vi "Data fgv.vi"(7 "Modes":T2, 8 "error in (no error)":errorcluster, 10 "Data":T1(array[cluster])) -> (0 "error out":errorcluster, 1 "Load?":bool, 2 "Position?":bool, 3 "appended array":dbl[][](array[numeric]), 4 "Data":bool)   [LabVIEW 2016]
uses:
  Controls/data modes.ctl
  <vilib>/gmath/NI_Gmath.lvlib
panel:
  out "x-y":dbl
  out "XY Graph 2":cluster{dbl[], "yi":dbl[]}[](graph)
  out "XY Graph":cluster{dbl[], "yi":dbl[]}[](graph)
  out "Waveform Graph 4":dbl[](graph)
  out "Waveform Graph 3":dbl[](graph)
  out "Waveform Graph 2":dbl[](graph)
  out "xi used 2":dbl[](array[numeric]) format="%_6g"
  out "Array 2":dbl[](array[numeric])
  out "Waveform Graph":dbl[](graph)
  out "xi used":dbl[](array[numeric]) format="%_6g"
  out "Array":dbl[](array[numeric])
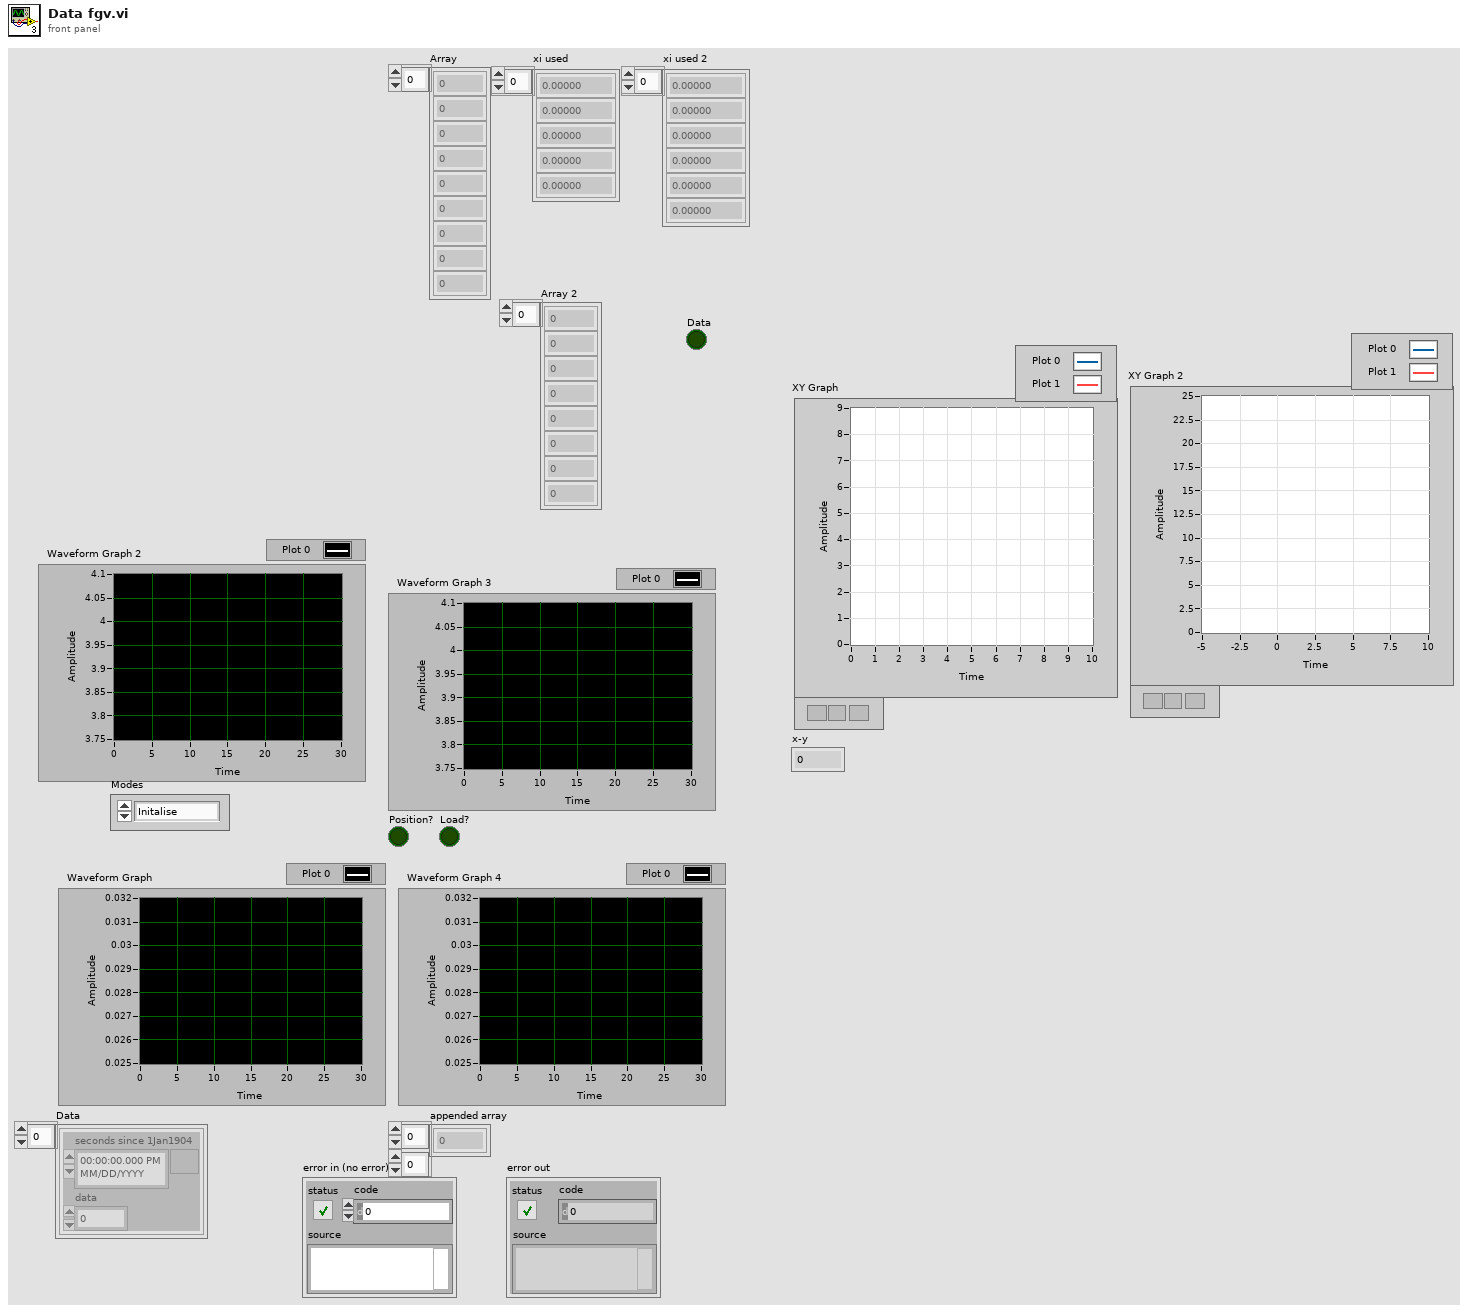
[diagram p1: front panel]
types:
  T1 = cluster{"seconds since 1Jan1904":timestamp, "data":dbl}[]
  T2 = typedef "data modes.ctl" = enum16{"Initalise", "Status", "Process", "Add load", "Add position"}
  T3 = cluster{"seconds since 1Jan1904":timestamp, "Numeric 2":dbl}[]
  T4 = cluster{"seconds since 1Jan1904":timestamp, "data":dbl}
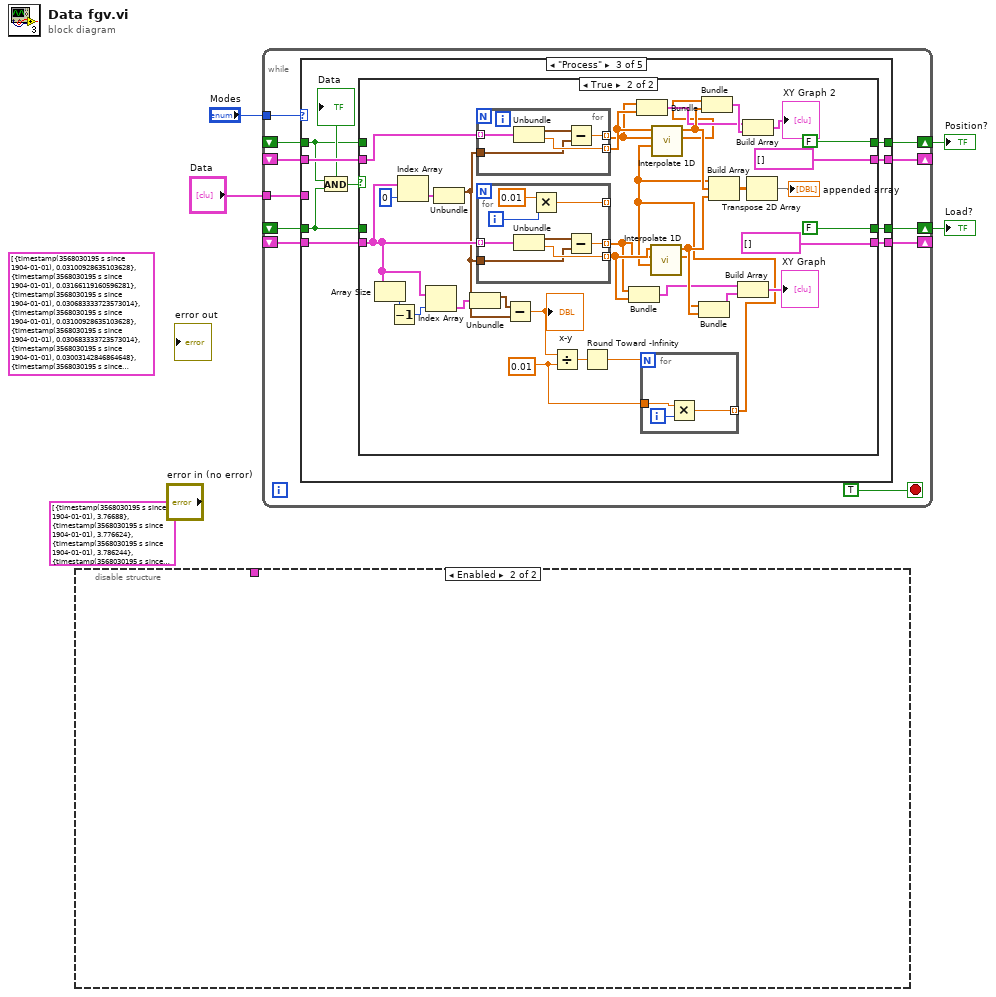
[diagram p0: block diagram]
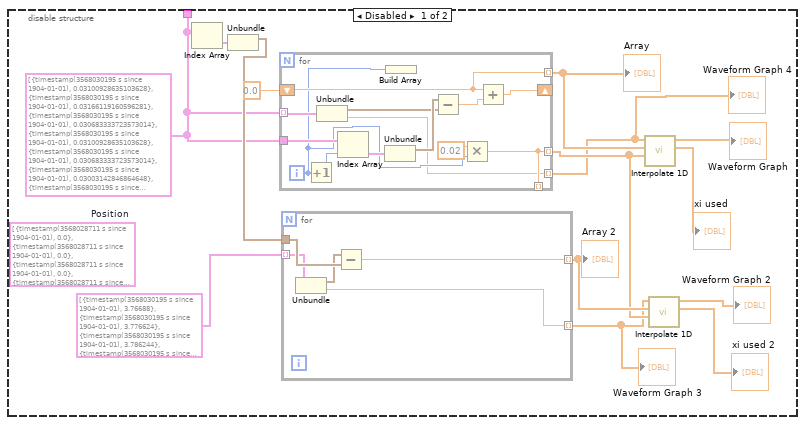
[diagram p2: hidden frame]
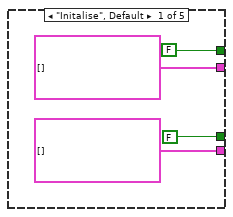
[diagram p3: hidden frame]
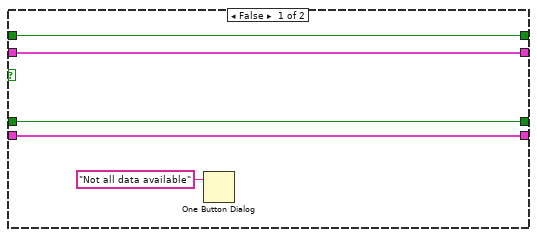
[diagram p5: hidden frame]
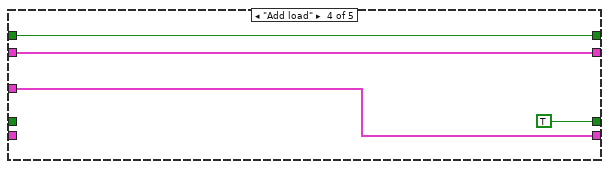
[diagram p6: hidden frame]
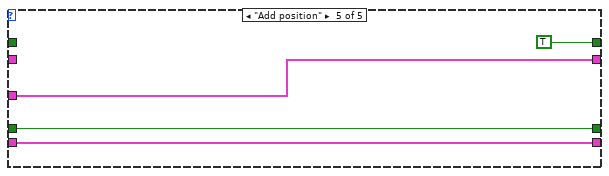
[diagram p7: hidden frame]
diagram:
  (unwired) T3 [{"seconds since 1Jan1904"=timestamp(3568030195.4029393 s since 1904-01-01), "Numeric 2"=3.76688}, {"seconds since 1Jan1904"=timestamp(3568030195.422031 s since 1904-01-01), "Numeric 2"=3.776624}, {"seconds since 1Jan1904"=timestamp(3568030195.441176 s since 1904-01-01), "Numeric 2"=3.786244}, {"seconds since 1Jan1904"=timestamp(3568030195.4632673 s since 1904-01-01), "Numeric 2"=3.796863}, {"seconds since 1Jan1904"=timestamp(3568030195.482293 s since 1904-01-01), "Numeric 2"=3.806608}, {"seconds since 1Jan1904"=timestamp(3568030195.501838 s since 1904-01-01), "Numeric 2"=3.816478}, {"seconds since 1Jan1904"=timestamp(3568030195.5218935 s since 1904-01-01), "Numeric 2"=3.826222}, {"seconds since 1Jan1904"=timestamp(3568030195.54296 s since 1904-01-01), "Numeric 2"=3.836841}, {"seconds since 1Jan1904"=timestamp(3568030195.5628576 s since 1904-01-01), "Numeric 2"=3.846836}, {"seconds since 1Jan1904"=timestamp(3568030195.582942 s since 1904-01-01), "Numeric 2"=3.85683}, {"seconds since 1Jan1904"=timestamp(3568030195.6025224 s since 1904-01-01), "Numeric 2"=3.866825}, {"seconds since 1Jan1904"=timestamp(3568030195.622336 s since 1904-01-01), "Numeric 2"=3.876445}, {"seconds since 1Jan1904"=timestamp(3568030195.642922 s since 1904-01-01), "Numeric 2"=3.886939}, {"seconds since 1Jan1904"=timestamp(3568030195.6669855 s since 1904-01-01), "Numeric 2"=3.898807}, {"seconds since 1Jan1904"=timestamp(3568030195.6822724 s since 1904-01-01), "Numeric 2"=3.906678}, {"seconds since 1Jan1904"=timestamp(3568030195.702325 s since 1904-01-01), "Numeric 2"=3.916672}, {"seconds since 1Jan1904"=timestamp(3568030195.72194 s since 1904-01-01), "Numeric 2"=3.926292}, {"seconds since 1Jan1904"=timestamp(3568030195.7419944 s since 1904-01-01), "Numeric 2"=3.936287}, {"seconds since 1Jan1904"=timestamp(3568030195.7638783 s since 1904-01-01), "Numeric 2"=3.947156}, {"seconds since 1Jan1904"=timestamp(3568030195.7819915 s since 1904-01-01), "Numeric 2"=3.956276}, {"seconds since 1Jan1904"=timestamp(3568030195.8025956 s since 1904-01-01), "Numeric 2"=3.966645}, {"seconds since 1Jan1904"=timestamp(3568030195.8226495 s since 1904-01-01), "Numeric 2"=3.976515}, {"seconds since 1Jan1904"=timestamp(3568030195.842401 s since 1904-01-01), "Numeric 2"=3.986509}, {"seconds since 1Jan1904"=timestamp(3568030195.862955 s since 1904-01-01), "Numeric 2"=3.996629}, {"seconds since 1Jan1904"=timestamp(3568030195.88289 s since 1904-01-01), "Numeric 2"=4.006748}, {"seconds since 1Jan1904"=timestamp(3568030195.9019513 s since 1904-01-01), "Numeric 2"=4.016368}, {"seconds since 1Jan1904"=timestamp(3568030195.9225645 s since 1904-01-01), "Numeric 2"=4.026487}, {"seconds since 1Jan1904"=timestamp(3568030195.942545 s since 1904-01-01), "Numeric 2"=4.036732}, {"seconds since 1Jan1904"=timestamp(3568030195.9630976 s since 1904-01-01), "Numeric 2"=4.046851}, {"seconds since 1Jan1904"=timestamp(3568030195.98266 s since 1904-01-01), "Numeric 2"=4.056471}] ("Array 3")
  (unwired) T1 [{"seconds since 1Jan1904"=timestamp(3568030195.391982 s since 1904-01-01), "data"=0.03100928635103628}, {"seconds since 1Jan1904"=timestamp(3568030195.4114995 s since 1904-01-01), "data"=0.03166119160596281}, {"seconds since 1Jan1904"=timestamp(3568030195.4307785 s since 1904-01-01), "data"=0.030683333723573014}, {"seconds since 1Jan1904"=timestamp(3568030195.4522047 s since 1904-01-01), "data"=0.03100928635103628}, {"seconds since 1Jan1904"=timestamp(3568030195.4717565 s since 1904-01-01), "data"=0.030683333723573014}, {"seconds since 1Jan1904"=timestamp(3568030195.4913096 s since 1904-01-01), "data"=0.03003142846864648}, {"seconds since 1Jan1904"=timestamp(3568030195.5108614 s since 1904-01-01), "data"=0.029705475841183215}, {"seconds since 1Jan1904"=timestamp(3568030195.5319176 s since 1904-01-01), "data"=0.02937952321371995}, {"seconds since 1Jan1904"=timestamp(3568030195.5513153 s since 1904-01-01), "data"=0.030357381096109748}, {"seconds since 1Jan1904"=timestamp(3568030195.5719137 s since 1904-01-01), "data"=0.029705475841183215}, {"seconds since 1Jan1904"=timestamp(3568030195.591967 s since 1904-01-01), "data"=0.029705475841183215}, {"seconds since 1Jan1904"=timestamp(3568030195.611306 s since 1904-01-01), "data"=0.02937952321371995}, {"seconds since 1Jan1904"=timestamp(3568030195.631862 s since 1904-01-01), "data"=0.02840166533133015}, {"seconds since 1Jan1904"=timestamp(3568030195.6559243 s since 1904-01-01), "data"=0.02937952321371995}, {"seconds since 1Jan1904"=timestamp(3568030195.671742 s since 1904-01-01), "data"=0.028075712703866884}, {"seconds since 1Jan1904"=timestamp(3568030195.6917977 s since 1904-01-01), "data"=0.02840166533133015}, {"seconds since 1Jan1904"=timestamp(3568030195.711027 s since 1904-01-01), "data"=0.027749760076403618}, {"seconds since 1Jan1904"=timestamp(3568030195.730965 s since 1904-01-01), "data"=0.027749760076403618}, {"seconds since 1Jan1904"=timestamp(3568030195.7527533 s since 1904-01-01), "data"=0.027749760076403618}, {"seconds since 1Jan1904"=timestamp(3568030195.771014 s since 1904-01-01), "data"=0.027749760076403618}, {"seconds since 1Jan1904"=timestamp(3568030195.791657 s since 1904-01-01), "data"=0.02677190219401382}, {"seconds since 1Jan1904"=timestamp(3568030195.811627 s since 1904-01-01), "data"=0.027097854821477085}, {"seconds since 1Jan1904"=timestamp(3568030195.831372 s since 1904-01-01), "data"=0.027749760076403618}, {"seconds since 1Jan1904"=timestamp(3568030195.850931 s since 1904-01-01), "data"=0.026445949566550553}, {"seconds since 1Jan1904"=timestamp(3568030195.8718615 s since 1904-01-01), "data"=0.02677190219401382}, {"seconds since 1Jan1904"=timestamp(3568030195.8914046 s since 1904-01-01), "data"=0.026445949566550553}, {"seconds since 1Jan1904"=timestamp(3568030195.911457 s since 1904-01-01), "data"=0.026119996939087287}, {"seconds since 1Jan1904"=timestamp(3568030195.9320126 s since 1904-01-01), "data"=0.025142139056697488}, {"seconds since 1Jan1904"=timestamp(3568030195.952068 s since 1904-01-01), "data"=0.02579404431162402}, {"seconds since 1Jan1904"=timestamp(3568030195.9716344 s since 1904-01-01), "data"=0.025468091684160754}] ("appended array")
  n1 = disable-structure shown="Enabled" {
    disable-tunnel: [w5 _] -> _
    frame Disabled {
      (unwired) T3 [{"seconds since 1Jan1904"=timestamp(3568030195.4029393 s since 1904-01-01), "Numeric 2"=3.76688}, {"seconds since 1Jan1904"=timestamp(3568030195.422031 s since 1904-01-01), "Numeric 2"=3.776624}, {"seconds since 1Jan1904"=timestamp(3568030195.441176 s since 1904-01-01), "Numeric 2"=3.786244}, {"seconds since 1Jan1904"=timestamp(3568030195.4632673 s since 1904-01-01), "Numeric 2"=3.796863}, {"seconds since 1Jan1904"=timestamp(3568030195.482293 s since 1904-01-01), "Numeric 2"=3.806608}, {"seconds since 1Jan1904"=timestamp(3568030195.501838 s since 1904-01-01), "Numeric 2"=3.816478}, {"seconds since 1Jan1904"=timestamp(3568030195.5218935 s since 1904-01-01), "Numeric 2"=3.826222}, {"seconds since 1Jan1904"=timestamp(3568030195.54296 s since 1904-01-01), "Numeric 2"=3.836841}, {"seconds since 1Jan1904"=timestamp(3568030195.5628576 s since 1904-01-01), "Numeric 2"=3.846836}, {"seconds since 1Jan1904"=timestamp(3568030195.582942 s since 1904-01-01), "Numeric 2"=3.85683}, {"seconds since 1Jan1904"=timestamp(3568030195.6025224 s since 1904-01-01), "Numeric 2"=3.866825}, {"seconds since 1Jan1904"=timestamp(3568030195.622336 s since 1904-01-01), "Numeric 2"=3.876445}, {"seconds since 1Jan1904"=timestamp(3568030195.642922 s since 1904-01-01), "Numeric 2"=3.886939}, {"seconds since 1Jan1904"=timestamp(3568030195.6669855 s since 1904-01-01), "Numeric 2"=3.898807}, {"seconds since 1Jan1904"=timestamp(3568030195.6822724 s since 1904-01-01), "Numeric 2"=3.906678}, {"seconds since 1Jan1904"=timestamp(3568030195.702325 s since 1904-01-01), "Numeric 2"=3.916672}, {"seconds since 1Jan1904"=timestamp(3568030195.72194 s since 1904-01-01), "Numeric 2"=3.926292}, {"seconds since 1Jan1904"=timestamp(3568030195.7419944 s since 1904-01-01), "Numeric 2"=3.936287}, {"seconds since 1Jan1904"=timestamp(3568030195.7638783 s since 1904-01-01), "Numeric 2"=3.947156}, {"seconds since 1Jan1904"=timestamp(3568030195.7819915 s since 1904-01-01), "Numeric 2"=3.956276}, {"seconds since 1Jan1904"=timestamp(3568030195.8025956 s since 1904-01-01), "Numeric 2"=3.966645}, {"seconds since 1Jan1904"=timestamp(3568030195.8226495 s since 1904-01-01), "Numeric 2"=3.976515}, {"seconds since 1Jan1904"=timestamp(3568030195.842401 s since 1904-01-01), "Numeric 2"=3.986509}, {"seconds since 1Jan1904"=timestamp(3568030195.862955 s since 1904-01-01), "Numeric 2"=3.996629}, {"seconds since 1Jan1904"=timestamp(3568030195.88289 s since 1904-01-01), "Numeric 2"=4.006748}, {"seconds since 1Jan1904"=timestamp(3568030195.9019513 s since 1904-01-01), "Numeric 2"=4.016368}, {"seconds since 1Jan1904"=timestamp(3568030195.9225645 s since 1904-01-01), "Numeric 2"=4.026487}, {"seconds since 1Jan1904"=timestamp(3568030195.942545 s since 1904-01-01), "Numeric 2"=4.036732}, {"seconds since 1Jan1904"=timestamp(3568030195.9630976 s since 1904-01-01), "Numeric 2"=4.046851}, {"seconds since 1Jan1904"=timestamp(3568030195.98266 s since 1904-01-01), "Numeric 2"=4.056471}] ("Array 3")
      (unwired) T3 [{"seconds since 1Jan1904"=timestamp(3568030195.4029393 s since 1904-01-01), "Numeric 2"=3.76688}, {"seconds since 1Jan1904"=timestamp(3568030195.422031 s since 1904-01-01), "Numeric 2"=3.776624}, {"seconds since 1Jan1904"=timestamp(3568030195.441176 s since 1904-01-01), "Numeric 2"=3.786244}, {"seconds since 1Jan1904"=timestamp(3568030195.4632673 s since 1904-01-01), "Numeric 2"=3.796863}, {"seconds since 1Jan1904"=timestamp(3568030195.482293 s since 1904-01-01), "Numeric 2"=3.806608}, {"seconds since 1Jan1904"=timestamp(3568030195.501838 s since 1904-01-01), "Numeric 2"=3.816478}, {"seconds since 1Jan1904"=timestamp(3568030195.5218935 s since 1904-01-01), "Numeric 2"=3.826222}, {"seconds since 1Jan1904"=timestamp(3568030195.54296 s since 1904-01-01), "Numeric 2"=3.836841}, {"seconds since 1Jan1904"=timestamp(3568030195.5628576 s since 1904-01-01), "Numeric 2"=3.846836}, {"seconds since 1Jan1904"=timestamp(3568030195.582942 s since 1904-01-01), "Numeric 2"=3.85683}, {"seconds since 1Jan1904"=timestamp(3568030195.6025224 s since 1904-01-01), "Numeric 2"=3.866825}, {"seconds since 1Jan1904"=timestamp(3568030195.622336 s since 1904-01-01), "Numeric 2"=3.876445}, {"seconds since 1Jan1904"=timestamp(3568030195.642922 s since 1904-01-01), "Numeric 2"=3.886939}, {"seconds since 1Jan1904"=timestamp(3568030195.6669855 s since 1904-01-01), "Numeric 2"=3.898807}, {"seconds since 1Jan1904"=timestamp(3568030195.6822724 s since 1904-01-01), "Numeric 2"=3.906678}, {"seconds since 1Jan1904"=timestamp(3568030195.702325 s since 1904-01-01), "Numeric 2"=3.916672}, {"seconds since 1Jan1904"=timestamp(3568030195.72194 s since 1904-01-01), "Numeric 2"=3.926292}, {"seconds since 1Jan1904"=timestamp(3568030195.7419944 s since 1904-01-01), "Numeric 2"=3.936287}, {"seconds since 1Jan1904"=timestamp(3568030195.7638783 s since 1904-01-01), "Numeric 2"=3.947156}, {"seconds since 1Jan1904"=timestamp(3568030195.7819915 s since 1904-01-01), "Numeric 2"=3.956276}, {"seconds since 1Jan1904"=timestamp(3568030195.8025956 s since 1904-01-01), "Numeric 2"=3.966645}, {"seconds since 1Jan1904"=timestamp(3568030195.8226495 s since 1904-01-01), "Numeric 2"=3.976515}, {"seconds since 1Jan1904"=timestamp(3568030195.842401 s since 1904-01-01), "Numeric 2"=3.986509}, {"seconds since 1Jan1904"=timestamp(3568030195.862955 s since 1904-01-01), "Numeric 2"=3.996629}, {"seconds since 1Jan1904"=timestamp(3568030195.88289 s since 1904-01-01), "Numeric 2"=4.006748}, {"seconds since 1Jan1904"=timestamp(3568030195.9019513 s since 1904-01-01), "Numeric 2"=4.016368}, {"seconds since 1Jan1904"=timestamp(3568030195.9225645 s since 1904-01-01), "Numeric 2"=4.026487}, {"seconds since 1Jan1904"=timestamp(3568030195.942545 s since 1904-01-01), "Numeric 2"=4.036732}, {"seconds since 1Jan1904"=timestamp(3568030195.9630976 s since 1904-01-01), "Numeric 2"=4.046851}, {"seconds since 1Jan1904"=timestamp(3568030195.98266 s since 1904-01-01), "Numeric 2"=4.056471}] ("Array 3")
      (unwired) T3 [{"seconds since 1Jan1904"=timestamp(3568030195.4029393 s since 1904-01-01), "Numeric 2"=3.76688}, {"seconds since 1Jan1904"=timestamp(3568030195.422031 s since 1904-01-01), "Numeric 2"=3.776624}, {"seconds since 1Jan1904"=timestamp(3568030195.441176 s since 1904-01-01), "Numeric 2"=3.786244}, {"seconds since 1Jan1904"=timestamp(3568030195.4632673 s since 1904-01-01), "Numeric 2"=3.796863}, {"seconds since 1Jan1904"=timestamp(3568030195.482293 s since 1904-01-01), "Numeric 2"=3.806608}, {"seconds since 1Jan1904"=timestamp(3568030195.501838 s since 1904-01-01), "Numeric 2"=3.816478}, {"seconds since 1Jan1904"=timestamp(3568030195.5218935 s since 1904-01-01), "Numeric 2"=3.826222}, {"seconds since 1Jan1904"=timestamp(3568030195.54296 s since 1904-01-01), "Numeric 2"=3.836841}, {"seconds since 1Jan1904"=timestamp(3568030195.5628576 s since 1904-01-01), "Numeric 2"=3.846836}, {"seconds since 1Jan1904"=timestamp(3568030195.582942 s since 1904-01-01), "Numeric 2"=3.85683}, {"seconds since 1Jan1904"=timestamp(3568030195.6025224 s since 1904-01-01), "Numeric 2"=3.866825}, {"seconds since 1Jan1904"=timestamp(3568030195.622336 s since 1904-01-01), "Numeric 2"=3.876445}, {"seconds since 1Jan1904"=timestamp(3568030195.642922 s since 1904-01-01), "Numeric 2"=3.886939}, {"seconds since 1Jan1904"=timestamp(3568030195.6669855 s since 1904-01-01), "Numeric 2"=3.898807}, {"seconds since 1Jan1904"=timestamp(3568030195.6822724 s since 1904-01-01), "Numeric 2"=3.906678}, {"seconds since 1Jan1904"=timestamp(3568030195.702325 s since 1904-01-01), "Numeric 2"=3.916672}, {"seconds since 1Jan1904"=timestamp(3568030195.72194 s since 1904-01-01), "Numeric 2"=3.926292}, {"seconds since 1Jan1904"=timestamp(3568030195.7419944 s since 1904-01-01), "Numeric 2"=3.936287}, {"seconds since 1Jan1904"=timestamp(3568030195.7638783 s since 1904-01-01), "Numeric 2"=3.947156}, {"seconds since 1Jan1904"=timestamp(3568030195.7819915 s since 1904-01-01), "Numeric 2"=3.956276}, {"seconds since 1Jan1904"=timestamp(3568030195.8025956 s since 1904-01-01), "Numeric 2"=3.966645}, {"seconds since 1Jan1904"=timestamp(3568030195.8226495 s since 1904-01-01), "Numeric 2"=3.976515}, {"seconds since 1Jan1904"=timestamp(3568030195.842401 s since 1904-01-01), "Numeric 2"=3.986509}, {"seconds since 1Jan1904"=timestamp(3568030195.862955 s since 1904-01-01), "Numeric 2"=3.996629}, {"seconds since 1Jan1904"=timestamp(3568030195.88289 s since 1904-01-01), "Numeric 2"=4.006748}, {"seconds since 1Jan1904"=timestamp(3568030195.9019513 s since 1904-01-01), "Numeric 2"=4.016368}, {"seconds since 1Jan1904"=timestamp(3568030195.9225645 s since 1904-01-01), "Numeric 2"=4.026487}, {"seconds since 1Jan1904"=timestamp(3568030195.942545 s since 1904-01-01), "Numeric 2"=4.036732}, {"seconds since 1Jan1904"=timestamp(3568030195.9630976 s since 1904-01-01), "Numeric 2"=4.046851}, {"seconds since 1Jan1904"=timestamp(3568030195.98266 s since 1904-01-01), "Numeric 2"=4.056471}] ("Array 3")
      (unwired) T3 [{"seconds since 1Jan1904"=timestamp(3568030195.4029393 s since 1904-01-01), "Numeric 2"=3.76688}, {"seconds since 1Jan1904"=timestamp(3568030195.422031 s since 1904-01-01), "Numeric 2"=3.776624}, {"seconds since 1Jan1904"=timestamp(3568030195.441176 s since 1904-01-01), "Numeric 2"=3.786244}, {"seconds since 1Jan1904"=timestamp(3568030195.4632673 s since 1904-01-01), "Numeric 2"=3.796863}, {"seconds since 1Jan1904"=timestamp(3568030195.482293 s since 1904-01-01), "Numeric 2"=3.806608}, {"seconds since 1Jan1904"=timestamp(3568030195.501838 s since 1904-01-01), "Numeric 2"=3.816478}, {"seconds since 1Jan1904"=timestamp(3568030195.5218935 s since 1904-01-01), "Numeric 2"=3.826222}, {"seconds since 1Jan1904"=timestamp(3568030195.54296 s since 1904-01-01), "Numeric 2"=3.836841}, {"seconds since 1Jan1904"=timestamp(3568030195.5628576 s since 1904-01-01), "Numeric 2"=3.846836}, {"seconds since 1Jan1904"=timestamp(3568030195.582942 s since 1904-01-01), "Numeric 2"=3.85683}, {"seconds since 1Jan1904"=timestamp(3568030195.6025224 s since 1904-01-01), "Numeric 2"=3.866825}, {"seconds since 1Jan1904"=timestamp(3568030195.622336 s since 1904-01-01), "Numeric 2"=3.876445}, {"seconds since 1Jan1904"=timestamp(3568030195.642922 s since 1904-01-01), "Numeric 2"=3.886939}, {"seconds since 1Jan1904"=timestamp(3568030195.6669855 s since 1904-01-01), "Numeric 2"=3.898807}, {"seconds since 1Jan1904"=timestamp(3568030195.6822724 s since 1904-01-01), "Numeric 2"=3.906678}, {"seconds since 1Jan1904"=timestamp(3568030195.702325 s since 1904-01-01), "Numeric 2"=3.916672}, {"seconds since 1Jan1904"=timestamp(3568030195.72194 s since 1904-01-01), "Numeric 2"=3.926292}, {"seconds since 1Jan1904"=timestamp(3568030195.7419944 s since 1904-01-01), "Numeric 2"=3.936287}, {"seconds since 1Jan1904"=timestamp(3568030195.7638783 s since 1904-01-01), "Numeric 2"=3.947156}, {"seconds since 1Jan1904"=timestamp(3568030195.7819915 s since 1904-01-01), "Numeric 2"=3.956276}, {"seconds since 1Jan1904"=timestamp(3568030195.8025956 s since 1904-01-01), "Numeric 2"=3.966645}, {"seconds since 1Jan1904"=timestamp(3568030195.8226495 s since 1904-01-01), "Numeric 2"=3.976515}, {"seconds since 1Jan1904"=timestamp(3568030195.842401 s since 1904-01-01), "Numeric 2"=3.986509}, {"seconds since 1Jan1904"=timestamp(3568030195.862955 s since 1904-01-01), "Numeric 2"=3.996629}, {"seconds since 1Jan1904"=timestamp(3568030195.88289 s since 1904-01-01), "Numeric 2"=4.006748}, {"seconds since 1Jan1904"=timestamp(3568030195.9019513 s since 1904-01-01), "Numeric 2"=4.016368}, {"seconds since 1Jan1904"=timestamp(3568030195.9225645 s since 1904-01-01), "Numeric 2"=4.026487}, {"seconds since 1Jan1904"=timestamp(3568030195.942545 s since 1904-01-01), "Numeric 2"=4.036732}, {"seconds since 1Jan1904"=timestamp(3568030195.9630976 s since 1904-01-01), "Numeric 2"=4.046851}, {"seconds since 1Jan1904"=timestamp(3568030195.98266 s since 1904-01-01), "Numeric 2"=4.056471}] ("Array 3")
      (unwired) T3 [{"seconds since 1Jan1904"=timestamp(3568030195.4029393 s since 1904-01-01), "Numeric 2"=3.76688}, {"seconds since 1Jan1904"=timestamp(3568030195.422031 s since 1904-01-01), "Numeric 2"=3.776624}, {"seconds since 1Jan1904"=timestamp(3568030195.441176 s since 1904-01-01), "Numeric 2"=3.786244}, {"seconds since 1Jan1904"=timestamp(3568030195.4632673 s since 1904-01-01), "Numeric 2"=3.796863}, {"seconds since 1Jan1904"=timestamp(3568030195.482293 s since 1904-01-01), "Numeric 2"=3.806608}, {"seconds since 1Jan1904"=timestamp(3568030195.501838 s since 1904-01-01), "Numeric 2"=3.816478}, {"seconds since 1Jan1904"=timestamp(3568030195.5218935 s since 1904-01-01), "Numeric 2"=3.826222}, {"seconds since 1Jan1904"=timestamp(3568030195.54296 s since 1904-01-01), "Numeric 2"=3.836841}, {"seconds since 1Jan1904"=timestamp(3568030195.5628576 s since 1904-01-01), "Numeric 2"=3.846836}, {"seconds since 1Jan1904"=timestamp(3568030195.582942 s since 1904-01-01), "Numeric 2"=3.85683}, {"seconds since 1Jan1904"=timestamp(3568030195.6025224 s since 1904-01-01), "Numeric 2"=3.866825}, {"seconds since 1Jan1904"=timestamp(3568030195.622336 s since 1904-01-01), "Numeric 2"=3.876445}, {"seconds since 1Jan1904"=timestamp(3568030195.642922 s since 1904-01-01), "Numeric 2"=3.886939}, {"seconds since 1Jan1904"=timestamp(3568030195.6669855 s since 1904-01-01), "Numeric 2"=3.898807}, {"seconds since 1Jan1904"=timestamp(3568030195.6822724 s since 1904-01-01), "Numeric 2"=3.906678}, {"seconds since 1Jan1904"=timestamp(3568030195.702325 s since 1904-01-01), "Numeric 2"=3.916672}, {"seconds since 1Jan1904"=timestamp(3568030195.72194 s since 1904-01-01), "Numeric 2"=3.926292}, {"seconds since 1Jan1904"=timestamp(3568030195.7419944 s since 1904-01-01), "Numeric 2"=3.936287}, {"seconds since 1Jan1904"=timestamp(3568030195.7638783 s since 1904-01-01), "Numeric 2"=3.947156}, {"seconds since 1Jan1904"=timestamp(3568030195.7819915 s since 1904-01-01), "Numeric 2"=3.956276}, {"seconds since 1Jan1904"=timestamp(3568030195.8025956 s since 1904-01-01), "Numeric 2"=3.966645}, {"seconds since 1Jan1904"=timestamp(3568030195.8226495 s since 1904-01-01), "Numeric 2"=3.976515}, {"seconds since 1Jan1904"=timestamp(3568030195.842401 s since 1904-01-01), "Numeric 2"=3.986509}, {"seconds since 1Jan1904"=timestamp(3568030195.862955 s since 1904-01-01), "Numeric 2"=3.996629}, {"seconds since 1Jan1904"=timestamp(3568030195.88289 s since 1904-01-01), "Numeric 2"=4.006748}, {"seconds since 1Jan1904"=timestamp(3568030195.9019513 s since 1904-01-01), "Numeric 2"=4.016368}, {"seconds since 1Jan1904"=timestamp(3568030195.9225645 s since 1904-01-01), "Numeric 2"=4.026487}, {"seconds since 1Jan1904"=timestamp(3568030195.942545 s since 1904-01-01), "Numeric 2"=4.036732}, {"seconds since 1Jan1904"=timestamp(3568030195.9630976 s since 1904-01-01), "Numeric 2"=4.046851}, {"seconds since 1Jan1904"=timestamp(3568030195.98266 s since 1904-01-01), "Numeric 2"=4.056471}] ("Array 3")
      w5 = T1 [{"seconds since 1Jan1904"=timestamp(3568030195.391982 s since 1904-01-01), "data"=0.03100928635103628}, {"seconds since 1Jan1904"=timestamp(3568030195.4114995 s since 1904-01-01), "data"=0.03166119160596281}, {"seconds since 1Jan1904"=timestamp(3568030195.4307785 s since 1904-01-01), "data"=0.030683333723573014}, {"seconds since 1Jan1904"=timestamp(3568030195.4522047 s since 1904-01-01), "data"=0.03100928635103628}, {"seconds since 1Jan1904"=timestamp(3568030195.4717565 s since 1904-01-01), "data"=0.030683333723573014}, {"seconds since 1Jan1904"=timestamp(3568030195.4913096 s since 1904-01-01), "data"=0.03003142846864648}, {"seconds since 1Jan1904"=timestamp(3568030195.5108614 s since 1904-01-01), "data"=0.029705475841183215}, {"seconds since 1Jan1904"=timestamp(3568030195.5319176 s since 1904-01-01), "data"=0.02937952321371995}, {"seconds since 1Jan1904"=timestamp(3568030195.5513153 s since 1904-01-01), "data"=0.030357381096109748}, {"seconds since 1Jan1904"=timestamp(3568030195.5719137 s since 1904-01-01), "data"=0.029705475841183215}, {"seconds since 1Jan1904"=timestamp(3568030195.591967 s since 1904-01-01), "data"=0.029705475841183215}, {"seconds since 1Jan1904"=timestamp(3568030195.611306 s since 1904-01-01), "data"=0.02937952321371995}, {"seconds since 1Jan1904"=timestamp(3568030195.631862 s since 1904-01-01), "data"=0.02840166533133015}, {"seconds since 1Jan1904"=timestamp(3568030195.6559243 s since 1904-01-01), "data"=0.02937952321371995}, {"seconds since 1Jan1904"=timestamp(3568030195.671742 s since 1904-01-01), "data"=0.028075712703866884}, {"seconds since 1Jan1904"=timestamp(3568030195.6917977 s since 1904-01-01), "data"=0.02840166533133015}, {"seconds since 1Jan1904"=timestamp(3568030195.711027 s since 1904-01-01), "data"=0.027749760076403618}, {"seconds since 1Jan1904"=timestamp(3568030195.730965 s since 1904-01-01), "data"=0.027749760076403618}, {"seconds since 1Jan1904"=timestamp(3568030195.7527533 s since 1904-01-01), "data"=0.027749760076403618}, {"seconds since 1Jan1904"=timestamp(3568030195.771014 s since 1904-01-01), "data"=0.027749760076403618}, {"seconds since 1Jan1904"=timestamp(3568030195.791657 s since 1904-01-01), "data"=0.02677190219401382}, {"seconds since 1Jan1904"=timestamp(3568030195.811627 s since 1904-01-01), "data"=0.027097854821477085}, {"seconds since 1Jan1904"=timestamp(3568030195.831372 s since 1904-01-01), "data"=0.027749760076403618}, {"seconds since 1Jan1904"=timestamp(3568030195.850931 s since 1904-01-01), "data"=0.026445949566550553}, {"seconds since 1Jan1904"=timestamp(3568030195.8718615 s since 1904-01-01), "data"=0.02677190219401382}, {"seconds since 1Jan1904"=timestamp(3568030195.8914046 s since 1904-01-01), "data"=0.026445949566550553}, {"seconds since 1Jan1904"=timestamp(3568030195.911457 s since 1904-01-01), "data"=0.026119996939087287}, {"seconds since 1Jan1904"=timestamp(3568030195.9320126 s since 1904-01-01), "data"=0.025142139056697488}, {"seconds since 1Jan1904"=timestamp(3568030195.952068 s since 1904-01-01), "data"=0.02579404431162402}, {"seconds since 1Jan1904"=timestamp(3568030195.9716344 s since 1904-01-01), "data"=0.025468091684160754}] ("appended array")
      (unwired) T3 [{"seconds since 1Jan1904"=timestamp(3568028711.3615117 s since 1904-01-01), "Numeric 2"=0.0}, {"seconds since 1Jan1904"=timestamp(3568028711.38202 s since 1904-01-01), "Numeric 2"=0.0}, {"seconds since 1Jan1904"=timestamp(3568028711.402072 s since 1904-01-01), "Numeric 2"=0.0}, {"seconds since 1Jan1904"=timestamp(3568028711.4226437 s since 1904-01-01), "Numeric 2"=0.0}, {"seconds since 1Jan1904"=timestamp(3568028711.442198 s since 1904-01-01), "Numeric 2"=0.0}, {"seconds since 1Jan1904"=timestamp(3568028711.461251 s since 1904-01-01), "Numeric 2"=0.0}, {"seconds since 1Jan1904"=timestamp(3568028711.4828105 s since 1904-01-01), "Numeric 2"=0.0}, {"seconds since 1Jan1904"=timestamp(3568028711.502207 s since 1904-01-01), "Numeric 2"=0.0}, {"seconds since 1Jan1904"=timestamp(3568028711.5223413 s since 1904-01-01), "Numeric 2"=0.0}, {"seconds since 1Jan1904"=timestamp(3568028711.542847 s since 1904-01-01), "Numeric 2"=0.0}, {"seconds since 1Jan1904"=timestamp(3568028711.561898 s since 1904-01-01), "Numeric 2"=0.0}, {"seconds since 1Jan1904"=timestamp(3568028711.58195 s since 1904-01-01), "Numeric 2"=0.0}, {"seconds since 1Jan1904"=timestamp(3568028711.6025076 s since 1904-01-01), "Numeric 2"=0.0}, {"seconds since 1Jan1904"=timestamp(3568028711.623597 s since 1904-01-01), "Numeric 2"=0.0}, {"seconds since 1Jan1904"=timestamp(3568028711.6426435 s since 1904-01-01), "Numeric 2"=0.0}, {"seconds since 1Jan1904"=timestamp(3568028711.662163 s since 1904-01-01), "Numeric 2"=0.0}, {"seconds since 1Jan1904"=timestamp(3568028711.6819606 s since 1904-01-01), "Numeric 2"=0.0}, {"seconds since 1Jan1904"=timestamp(3568028711.702017 s since 1904-01-01), "Numeric 2"=0.0}, {"seconds since 1Jan1904"=timestamp(3568028711.7225213 s since 1904-01-01), "Numeric 2"=0.0}, {"seconds since 1Jan1904"=timestamp(3568028711.743164 s since 1904-01-01), "Numeric 2"=0.0}, {"seconds since 1Jan1904"=timestamp(3568028711.762731 s since 1904-01-01), "Numeric 2"=0.0}, {"seconds since 1Jan1904"=timestamp(3568028711.781278 s since 1904-01-01), "Numeric 2"=0.0}, {"seconds since 1Jan1904"=timestamp(3568028711.8018117 s since 1904-01-01), "Numeric 2"=0.0}, {"seconds since 1Jan1904"=timestamp(3568028711.82237 s since 1904-01-01), "Numeric 2"=0.0}, {"seconds since 1Jan1904"=timestamp(3568028711.8418393 s since 1904-01-01), "Numeric 2"=0.0}, {"seconds since 1Jan1904"=timestamp(3568028711.8622947 s since 1904-01-01), "Numeric 2"=0.0}, {"seconds since 1Jan1904"=timestamp(3568028711.8836417 s since 1904-01-01), "Numeric 2"=0.0}, {"seconds since 1Jan1904"=timestamp(3568028711.903713 s since 1904-01-01), "Numeric 2"=0.0}, {"seconds since 1Jan1904"=timestamp(3568028711.921743 s since 1904-01-01), "Numeric 2"=0.0}, {"seconds since 1Jan1904"=timestamp(3568028711.942297 s since 1904-01-01), "Numeric 2"=0.0}]  # Position
      n2 = Index Array(array=w5) -> (element=w17:T4)  [unwired: 1 in]
      n3 = Unbundle(w17) -> ("seconds since 1Jan1904"=w13:timestamp)  [unwired: 1 out]
      n4 = for {
        tunnel: w5 -> [w34] mode=indexing
        shift-right: [w30] -> _
        shift-left: 0.0 -> [w29]
        tunnel: w5 -> [w36]
        tunnel: [w29] -> w16 mode=indexing
        tunnel: [w24] -> w6 mode=indexing
        tunnel: [w27] -> w11 mode=indexing
        tunnel: [w27] -> _ mode=indexing
        i -> [w25]
        n5 = Increment(x=w25) -> (x+1=w35:i32)
        n6 = Unbundle(w34) -> ("seconds since 1Jan1904"=w31:timestamp, "data"=w24:dbl)
        n7 = Index Array(array=w36, index=w35) -> (element=w33:T4)
        n8 = Unbundle(w33) -> ("seconds since 1Jan1904"=w32:timestamp)  [unwired: 1 out]
        n9 = Build Array(w25) -> ()  [unwired: 1 out]
        n10 = Subtract(x=w32, y=w31) -> (x-y=w26:dbl)
        n11 = Multiply(x=0.02, y=w25) -> (x*y=w27:dbl)
        n12 = Add(x=w29, y=w26) -> (x+y=w30:dbl)
      }
      "Array" <- w16
      "Waveform Graph 4" <- w6
      n13 = for {
        tunnel: T3 [{"seconds since 1Jan1904"=timestamp(3568030195.4029393 s since 1904-01-01), "Numeric 2"=3.76688}, {"seconds since 1Jan1904"=timestamp(3568030195.422031 s since 1904-01-01), "Numeric 2"=3.776624}, {"seconds since 1Jan1904"=timestamp(3568030195.441176 s since 1904-01-01), "Numeric 2"=3.786244}, {"seconds since 1Jan1904"=timestamp(3568030195.4632673 s since 1904-01-01), "Numeric 2"=3.796863}, {"seconds since 1Jan1904"=timestamp(3568030195.482293 s since 1904-01-01), "Numeric 2"=3.806608}, {"seconds since 1Jan1904"=timestamp(3568030195.501838 s since 1904-01-01), "Numeric 2"=3.816478}, {"seconds since 1Jan1904"=timestamp(3568030195.5218935 s since 1904-01-01), "Numeric 2"=3.826222}, {"seconds since 1Jan1904"=timestamp(3568030195.54296 s since 1904-01-01), "Numeric 2"=3.836841}, {"seconds since 1Jan1904"=timestamp(3568030195.5628576 s since 1904-01-01), "Numeric 2"=3.846836}, {"seconds since 1Jan1904"=timestamp(3568030195.582942 s since 1904-01-01), "Numeric 2"=3.85683}, {"seconds since 1Jan1904"=timestamp(3568030195.6025224 s since 1904-01-01), "Numeric 2"=3.866825}, {"seconds since 1Jan1904"=timestamp(3568030195.622336 s since 1904-01-01), "Numeric 2"=3.876445}, {"seconds since 1Jan1904"=timestamp(3568030195.642922 s since 1904-01-01), "Numeric 2"=3.886939}, {"seconds since 1Jan1904"=timestamp(3568030195.6669855 s since 1904-01-01), "Numeric 2"=3.898807}, {"seconds since 1Jan1904"=timestamp(3568030195.6822724 s since 1904-01-01), "Numeric 2"=3.906678}, {"seconds since 1Jan1904"=timestamp(3568030195.702325 s since 1904-01-01), "Numeric 2"=3.916672}, {"seconds since 1Jan1904"=timestamp(3568030195.72194 s since 1904-01-01), "Numeric 2"=3.926292}, {"seconds since 1Jan1904"=timestamp(3568030195.7419944 s since 1904-01-01), "Numeric 2"=3.936287}, {"seconds since 1Jan1904"=timestamp(3568030195.7638783 s since 1904-01-01), "Numeric 2"=3.947156}, {"seconds since 1Jan1904"=timestamp(3568030195.7819915 s since 1904-01-01), "Numeric 2"=3.956276}, {"seconds since 1Jan1904"=timestamp(3568030195.8025956 s since 1904-01-01), "Numeric 2"=3.966645}, {"seconds since 1Jan1904"=timestamp(3568030195.8226495 s since 1904-01-01), "Numeric 2"=3.976515}, {"seconds since 1Jan1904"=timestamp(3568030195.842401 s since 1904-01-01), "Numeric 2"=3.986509}, {"seconds since 1Jan1904"=timestamp(3568030195.862955 s since 1904-01-01), "Numeric 2"=3.996629}, {"seconds since 1Jan1904"=timestamp(3568030195.88289 s since 1904-01-01), "Numeric 2"=4.006748}, {"seconds since 1Jan1904"=timestamp(3568030195.9019513 s since 1904-01-01), "Numeric 2"=4.016368}, {"seconds since 1Jan1904"=timestamp(3568030195.9225645 s since 1904-01-01), "Numeric 2"=4.026487}, {"seconds since 1Jan1904"=timestamp(3568030195.942545 s since 1904-01-01), "Numeric 2"=4.036732}, {"seconds since 1Jan1904"=timestamp(3568030195.9630976 s since 1904-01-01), "Numeric 2"=4.046851}, {"seconds since 1Jan1904"=timestamp(3568030195.98266 s since 1904-01-01), "Numeric 2"=4.056471}] ("Array 3") -> [w22] mode=indexing
        tunnel: w13 -> [w23]
        tunnel: [w20] -> w12 mode=indexing
        tunnel: [w19] -> w8 mode=indexing
        n14 = Unbundle(w22) -> ("seconds since 1Jan1904"=w21:timestamp, "Numeric 2"=w19:dbl)
        n15 = Subtract(x=w21, y=w23) -> (x-y=w20:dbl)
      }
      "Array 2" <- w12
      "Waveform Graph 3" <- w8
      n16 = call <vilib>:"Interpolate 1D.vi"("xi"=w11, "X"=w16, "Y"=w6) -> ("xi used"=→"xi used":dbl[], "yi"=→"Waveform Graph":dbl[])  [unwired: 6 in, 1 out]
      n17 = call <vilib>:"Interpolate 1D.vi"("xi"=w11, "X"=w12, "Y"=w8) -> ("xi used"=→"xi used 2":dbl[], "yi"=→"Waveform Graph 2":dbl[])  [unwired: 6 in, 1 out]
    }
    frame Enabled {
    }
  }
  n18 = while {
    tunnel: "Modes" -> [w46]
    shift-right: [w44] -> _
    shift-left: _ -> [w45]
    shift-right: [w43] -> w3
    shift-left: _ -> [w42]
    shift-right: [w39] -> _
    shift-left: _ -> [w40]
    shift-right: [w38] -> w2
    shift-left: _ -> [w41]
    tunnel: "Data" -> [w37]
    stop <- TRUE stop-if-true
    n19 = case shown="\"Process\"" w46 {
      tunnel: w45 -> [_ w55 w63 w121 _]
      tunnel: [T1 [] ("appended array") w55 w57 w121 w127] -> w44
      tunnel: [FALSE w54 w56 w120 TRUE] -> w43
      tunnel: w42 -> [_ w54 w58 w120 _]
      tunnel: w41 -> [_ w52 w60 _ w125]
      tunnel: w40 -> [_ w53 w64 _ w124]
      tunnel: [T1 [] ("appended array") w53 w61 w122 w124] -> w39
      tunnel: [FALSE w52 w59 TRUE w125] -> w38
      tunnel: w37 -> [_ _ _ w122 w127]
      frame "Initalise", Default {
      }
      frame "Status" {
      }
      frame "Process" {
        n20 = And(x=w58, y=w60) -> (x .and. y?=w62:bool)
        "Data" <- w62
        n21 = case shown="True" w62 {
          tunnel: w64 -> [w68 w78]
          tunnel: w63 -> [w66 w101]
          tunnel: [w68 T1 [] ("appended array")] -> w61
          tunnel: w60 -> [w67 _]
          tunnel: [w67 FALSE] -> w59
          tunnel: w58 -> [w65 _]
          tunnel: [w66 T1 [] ("Data")] -> w57
          tunnel: [w65 FALSE] -> w56
          frame False {
            n22 = One Button Dialog(message="Not all data available") -> ()  [unwired: 1 in, 1 out]
          }
          frame True {
            w71 = 0.01
            n23 = Array Size(array=w78) -> (size(s)=w79:i32)
            n24 = Decrement(x=w79) -> (x-1=w80:i32)
            n25 = Index Array(array=w78, index=0) -> (element=w102:T4)
            n26 = Index Array(array=w78, index=w80) -> (element=w77:T4)
            n27 = Unbundle(w102) -> ("seconds since 1Jan1904"=w75:timestamp)  [unwired: 1 out]
            n28 = Unbundle(w77) -> ("seconds since 1Jan1904"=w76:timestamp)  [unwired: 1 out]
            n29 = for {
              tunnel: w101 -> [w111] mode=indexing
              tunnel: [w110] -> w90 mode=indexing
              tunnel: w75 -> [w108]
              tunnel: [w107] -> w89 mode=indexing
              n30 = Unbundle(w111) -> ("seconds since 1Jan1904"=w109:timestamp, "data"=w110:dbl)
              n31 = Subtract(x=w109, y=w108) -> (x-y=w107:dbl)
            }
            n32 = for {
              tunnel: w78 -> [w119] mode=indexing
              tunnel: [w115] -> w96 mode=indexing
              tunnel: [w117] -> _ mode=indexing
              tunnel: w75 -> [w113]
              tunnel: [w112] -> w94 mode=indexing
              i -> [w116]
              n33 = Unbundle(w119) -> ("seconds since 1Jan1904"=w114:timestamp, "data"=w115:dbl)
              n34 = Multiply(x=0.01, y=w116) -> (x*y=w117:dbl)
              n35 = Subtract(x=w114, y=w113) -> (x-y=w112:dbl)
            }
            n36 = Subtract(x=w76, y=w75) -> (x-y=w74:dbl)
            "x-y" <- w74
            n37 = Divide(x=w74, y=w71) -> (x/y=w73:dbl)
            n38 = Round Toward -Infinity(1:w73) -> (0:w72:dbl)
            n39 = Bundle(w94, w96) -> (w93:cluster{dbl[], dbl[]})  [unwired: 1 in]
            n40 = Bundle(w89, w90) -> (w86:cluster{dbl[], dbl[]})  [unwired: 1 in]
            n41 = for {
              N: w72 -> [_]
              tunnel: w71 -> [w105]
              tunnel: [w104] -> w70 mode=indexing
              i -> [w106]
              n42 = Multiply(x=w105, y=w106) -> (x*y=w104:dbl)
            }
            n43 = call <vilib>:"Interpolate 1D.vi"("xi"=w70, "X"=w94, "Y"=w96) -> ("xi used"=w84:dbl[], "yi"=w95:dbl[])  [unwired: 6 in, 1 out]
            n44 = call <vilib>:"Interpolate 1D.vi"("xi"=w70, "X"=w89, "Y"=w90) -> ("xi used"=w83:dbl[], "yi"=w88:dbl[])  [unwired: 6 in, 1 out]
            n45 = Bundle("xi used"=w84, "yi"=w95) -> (w92:cluster{"xi used":dbl[], "yi":dbl[]})  [unwired: 1 in]
            n46 = Bundle("xi used"=w83, "yi"=w88) -> (w87:cluster{"xi used":dbl[], "yi":dbl[]})  [unwired: 1 in]
            n47 = Build Array(w70, w88, w95) -> (w82:dbl[][])
            n48 = Build Array(w93, w92) -> (→"XY Graph":cluster{"xi used":dbl[], "yi":dbl[]}[])
            n49 = Build Array(w86, w87) -> (→"XY Graph 2":cluster{"xi used":dbl[], "yi":dbl[]}[])
            n50 = Transpose 2D Array(2D array=w82) -> (transposed array=→"appended array":dbl[][])
          }
        }
      }
      frame "Add load" {
      }
      frame "Add position" {
      }
    }
  }
  "Position?" <- w3
  "Load?" <- w2
